vi "control_disable_status.vi"(10 "control":refnum<vi>, 11 "status":bool) -> ()   [LabVIEW 2016, in "MotionControl_UFO_3DOF.lvlib"]
uses:
  <userlib>/MotionControl_UFO_3DOF/MotionControl_UFO_3DOF.lvlib
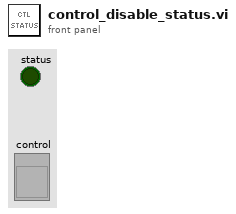
[diagram p1: front panel]
types:
  T1 = enum8{"Enabled", "Disabled", "Disabled and Grayed Out"}
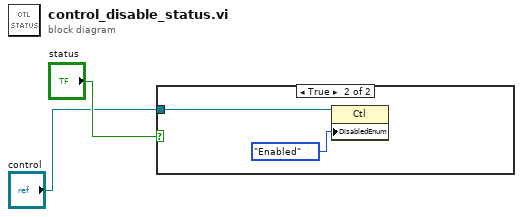
[diagram p0: block diagram]
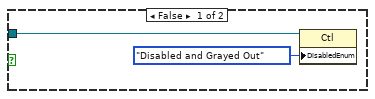
[diagram p2: hidden frame]
diagram:
  n1 = case shown="True" "status" {
    tunnel: "control" -> [w4 w6]
    frame False {
      n2 = property class="Ctl"(reference=w4, "DisabledEnum"=T1."Disabled and Grayed Out" ("禁用")) -> ()  [unwired: 1 in, 2 out]
    }
    frame True {
      n3 = property class="Ctl"(reference=w6, "DisabledEnum"=T1."Enabled" ("禁用")) -> ()  [unwired: 1 in, 2 out]
    }
  }
